vi "Configure IIC Trigger.vi"(4 "pattern data (0)":i32 caption="Pattern Data (0)", 5 "iic condition (Start Condition)":i32(ring) caption="IIC Condition (Start Condition)" items=["Start Condition", "Stop Condition", "Frame Read 7", "Frame Write 7", "Frame Write 10", "EEPROM Data Read", "Missing Acknowledge", "Restart"], 6 "device address (0)":i32 caption="Device Address (0)", 7 "trigger level (0.0 V)":dbl caption="Trigger Level (0.0 V)" format="%^.2e", 8 "error in (no error)":errorcluster {"code" format="%.0x"}, 9 "Serial Clock (Channel 1)":string(combo)="CHAN1", 10 "Serial Data (Channel 2)":string(combo)="CHAN2", 11 "VISA Resource Name":refnum<visa-resource-name>) -> (0 "error out":errorcluster {"code" format="%.0x"}, 3 "VISA Resource Name Out":refnum<visa-resource-name>)   [LabVIEW 2011, in "Agilent 546XX Series.lvlib"]
doc: "This VI configures the trigger level, serial data, serial clock, trigger condition, device address and data pattern for the IIC trigger.\n\nNote: This VI affects instrument behavior only if the trigger type is set to IIC Trigger. Call the ag546xx Configure Trigger and ag546xx Configure Trigger Coupling VIs to set the trigger type and trigger coupling before calling this VI."
uses:
  Agilent 546XX Series.lvlib
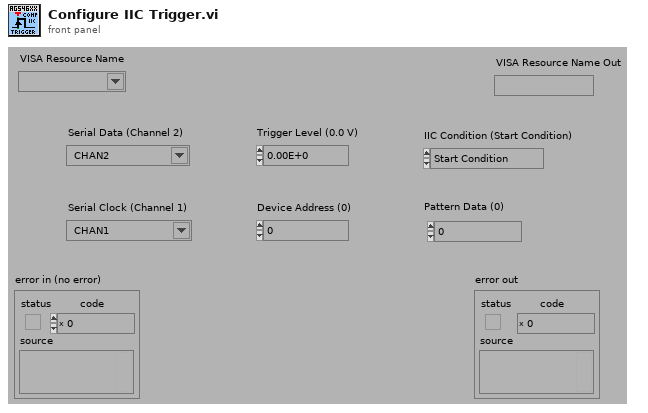
[diagram p1: front panel]
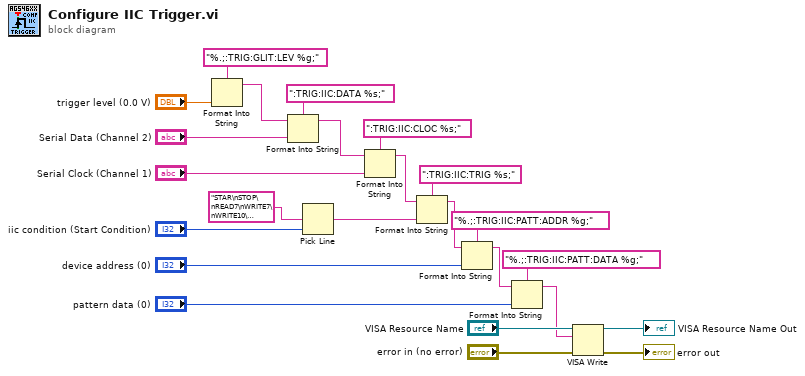
[diagram p0: block diagram]
diagram:
  n1 = Format Into String(format string="%.;:TRIG:GLIT:LEV %g;", "trigger level (0.0 V)") -> (resulting string=w17:string)  [unwired: 2 in, 1 out]
  n2 = Format Into String(format string=":TRIG:IIC:DATA %s;", initial string=w17, "Serial Data (Channel 2)") -> (resulting string=w15:string)  [unwired: 1 in, 1 out]
  n3 = Pick Line(multi-line string="STAR\nSTOP\nREAD7\nWRITE7\nWRITE10\nREADE\nNACK\nREST", line index="iic condition (Start Condition)") -> (output string=w11:string)  [unwired: 1 in]
  n4 = Format Into String(format string=":TRIG:IIC:CLOC %s;", initial string=w15, "Serial Clock (Channel 1)") -> (resulting string=w12:string)  [unwired: 1 in, 1 out]
  n5 = Format Into String(format string=":TRIG:IIC:TRIG %s;", initial string=w12, w11) -> (resulting string=w1:string)  [unwired: 1 in, 1 out]
  n6 = Format Into String(format string="%.;:TRIG:IIC:PATT:ADDR %g;", initial string=w1, "device address (0)") -> (resulting string=w6:string)  [unwired: 1 in, 1 out]
  n7 = Format Into String(format string="%.;:TRIG:IIC:PATT:DATA %g;", initial string=w6, "pattern data (0)") -> (resulting string=w3:string)  [unwired: 1 in, 1 out]
  n8 = VISA Write(VISA resource name="VISA Resource Name", write buffer=w3, error in (no error)="error in (no error)") -> (VISA resource name out=→"VISA Resource Name Out":refnum<visa-resource-name>, error out=→"error out":errorcluster)  [unwired: 1 out]
